vi "NaN suchen und mit altem Wert ersetzen.vi"(8 "Alte Messdaten":sgl[](array[numeric]), 11 "Neue Messdaten":sgl[](array[numeric])) -> (3 "Messdaten":sgl[](array[numeric]))   [LabVIEW 2020, in "Messdaten.lvlib"]
uses:
  Messdaten.lvlib
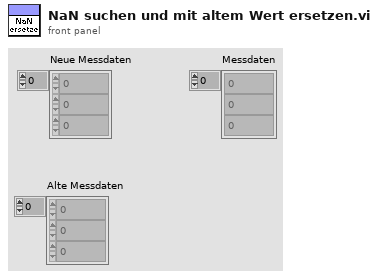
[diagram p1: front panel]
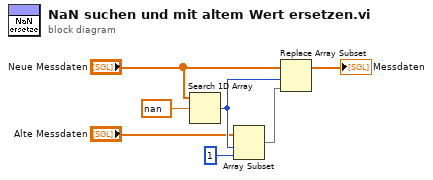
[diagram p0: block diagram]
diagram:
  n1 = Search 1D Array(1D array="Neue Messdaten", element=sgl nan ("Element")) -> (index of element=w6:i32)  [unwired: 1 in]
  n2 = Array Subset(array="Alte Messdaten", index=w6, length=1 ("Länge")) -> (w4:sgl[])
  n3 = Replace Array Subset(array="Neue Messdaten", new element=w4, index=w6) -> (→"Messdaten":sgl[])
